vi "Read from File Globals and Write to TSM.vi"(0 "TSM context":T1, 5 "Sequence Ref In":refnum<k7>) -> (15 "error out":errorcluster)   [LabVIEW 2019]
uses:
  <vilib>/NI_TestStand_SemiconductorModule/NI_TestStand_Semiconductor_Module.lvlibp/PinMap/General/SemiconductorModuleContext.ctl
  <vilib>/NI_TestStand_SemiconductorModule/NI_TestStand_Semiconductor_Module.lvlibp
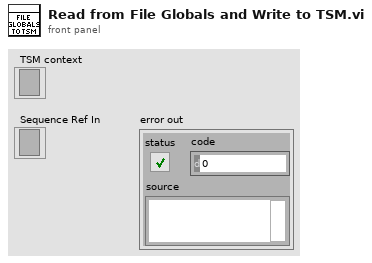
[diagram p1: front panel]
types:
  T1 = typedef "NI_TestStand_Semiconductor_Module.lvlibp/SemiconductorModuleContext.ctl" = refnum<k7>
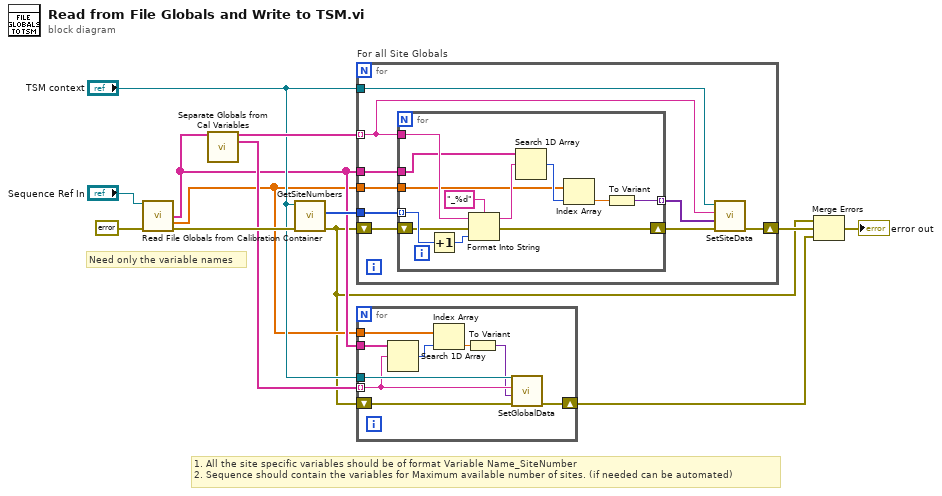
[diagram p0: block diagram]
diagram:
  # "1. All the site specific variables should be of format Variable Name_SiteNumber\n2. Sequence should contain the variables for Maximum available number of sites. (if needed can be automated)"
  # "Need only the variable names"
  n1 = call "Read File Globals from Calibration Container.vi"("Sequence Ref In"="Sequence Ref In", "error in"=errorcluster {"status"=FALSE, "code"=0, "source"=""} ("error in (no error)")) -> ("Calibration Variables"=w6:string[], "Values"=w5:dbl[], "error out"=w11:errorcluster)  [unwired: 8 in, 3 out]
  n2 = call "Separate Globals from Cal Variables.vi"("Calibration Variables"=w6) -> ("Site Globals"=w9:string[], "Globals"=w7:string[])  [unwired: 13 in]
  n3 = call <vilib>:"GetSiteNumbers.vi"("error in (no error)"=w11, "Semiconductor Module Context"="TSM context") -> ("error out"=w1:errorcluster, "Site Numbers"=w10:i32[])  [unwired: 6 in, 2 out]
  n4 = for "For all Site Globals" {
    tunnel: w10 -> [w22]
    tunnel: w5 -> [w20]
    tunnel: w9 -> [w17] mode=indexing
    tunnel: w6 -> [w21]
    tunnel: "TSM context" -> [w18]
    shift-right: [w16] -> w4
    shift-left: w1 -> [w15]
    n5 = for {
      shift-right: [w23] -> w19
      shift-left: w15 -> [w24]
      tunnel: w22 -> [w33] mode=indexing
      tunnel: w17 -> [w34]
      tunnel: w21 -> [w31]
      tunnel: w20 -> [w28]
      tunnel: [w25] -> w14 mode=indexing
      n6 = Increment(x=w33) -> (x+1=w26:i32)
      n7 = Format Into String(format string="_%d", initial string=w34, error in=w24, w26) -> (resulting string=w30:string, error out=w23:errorcluster)
      n8 = Search 1D Array(1D array=w31, element=w30) -> (index of element=w29:i32)  [unwired: 1 in]
      n9 = Index Array(array=w28, index=w29) -> (element=w27:dbl)
      n10 = To Variant(anything=w27) -> (Variant=w25:variant)
    }
    n11 = call <vilib>:"SetSiteData.vi"("error in (no error)"=w19, "Site Data"=w14, "Data Id"=w17, "Semiconductor Module Context"=w18) -> ("error out"=w16:errorcluster)  [unwired: 5 in, 1 out]
  }
  n12 = for {
    tunnel: "TSM context" -> [w43]
    tunnel: w7 -> [w40] mode=indexing
    tunnel: w6 -> [w41]
    tunnel: w5 -> [w38]
    shift-right: [w35] -> w3
    shift-left: w1 -> [w42]
    n13 = Search 1D Array(1D array=w41, element=w40) -> (index of element=w39:i32)  [unwired: 1 in]
    n14 = Index Array(array=w38, index=w39) -> (element=w37:dbl)
    n15 = To Variant(anything=w37) -> (Variant=w36:variant)
    n16 = call <vilib>:"SetGlobalData.vi"("error in (no error)"=w42, "Data"=w36, "Data Id"=w40, "Semiconductor Module Context"=w43) -> ("error out"=w35:errorcluster)  [unwired: 5 in, 1 out]
  }
  n17 = Merge Errors(w1, w4, w3) -> (→"error out":errorcluster)
